vi "Actor Core.vi"(8 "error in":errorcluster, 11 "New Event UI in":refnum<class "New Event UI.lvclass">) -> (0 "error out":errorcluster, 3 "Actor out":refnum<class "Actor.lvclass">)   [LabVIEW 2019, in "New Event UI.lvlib" / "New Event UI.lvclass"]
doc: "(<B>Filename</B>: Actor Framework.lvlib:Actor.lvclass:Actor Core.vi)\n\nReceives messages to the actor, reacts to them, and initiates any error handling that may shut the actor down.\n\nDescendant classes may override this VI to append parallel tasks for the actor to complete while it handles messages. Overrides use the Call Parent Method node."
uses:
  New Event UI.lvclass
  <vilib>/ActorFramework/Actor/Actor.lvclass
  UI Controller/UI Controller/UI Controller.lvclass
  UI Controller/UI Controller Messages/Create New Event Msg/Create New Event Msg.lvclass
  C:/GIT/Event-Diplom/Source/Event Diplom NI-AF/UI Controller/UI Controller/UI Controller.lvclass
  C:/Program Files (x86)/National Instruments/LabVIEW 2019/vi.lib/ActorFramework/Actor/Actor.lvclass
  <vilib>/ActorFramework/Stop Msg/Stop Msg.lvclass
  <vilib>/GPower/UI/Library/GP UI.lvlib
panel:
  in  "Cancel Button":bool
  in  "OK Button":bool
  in  "Member Data File Path":path
  in  "Description":string
  in  "Event Name":string
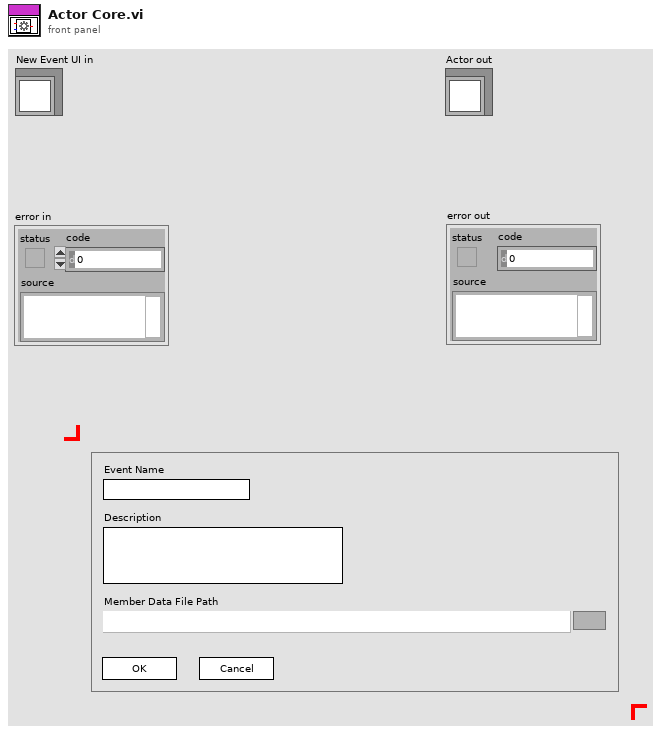
[diagram p1: front panel]
types:
  T1 = cluster{"Event Name":string, "Description":string, "Member Data File Path":path}
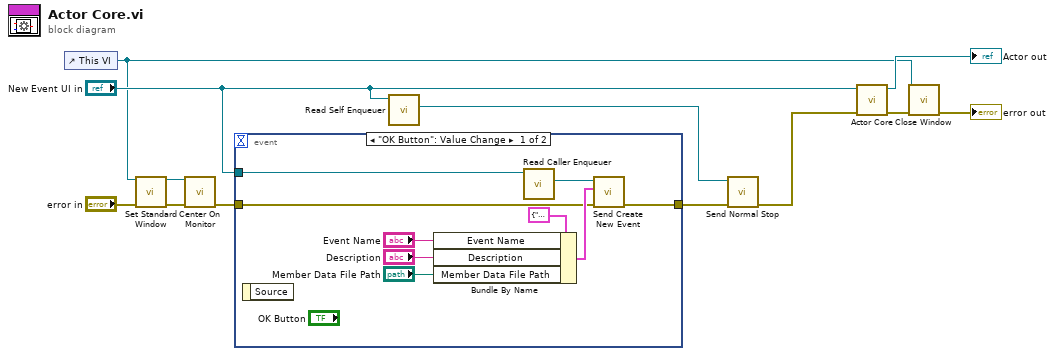
[diagram p0: block diagram]
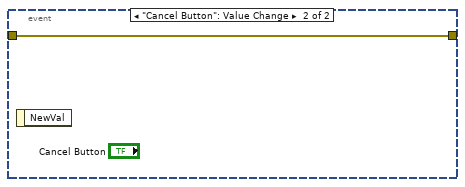
[diagram p2: hidden frame]
diagram:
  n1 = control-ref of="This VI"() -> (w3:refnum<vi>)
  n2 = call <vilib>:"Set Standard Window.vi"("VI Refnum"=w3, "Error in"="error in") -> ("Error out"=w6:errorcluster)  [unwired: 13 in]
  n3 = call <vilib>:"Center On Monitor.vi"("VI Refnum"=w3, "Error in"=w6) -> ("Error out"=w1:errorcluster)  [unwired: 13 in]
  n4 = event shown="[0] \"OK Button\": Value Change" {
    selector: _ -> [_ _]
    dyn-events: _ -> [_ _]
    timeout: _ -> [_ _]
    tunnel: "New Event UI in" -> [w20 _]
    tunnel: [w13 w21] -> w9
    tunnel: w1 -> [w12 w21]
    event "OK Button": Value Change {
      n5 = event-data() -> ()  [unwired: 1 in, 1 out]
      n6 = Bundle By Name(cluster=T1 {"Event Name"="", "Description"="", "Member Data File Path"=path ""} ("Event"), "Event Name"="Event Name", "Description"="Description", "Member Data File Path"="Member Data File Path") -> (w14:T1)
      n7 = call <vilib>:"Read Caller Enqueuer.vi"("Actor"=w20) -> ("Caller Enqueuer"=w19:refnum<class "Message Enqueuer.lvclass">)  [unwired: 10 in]
      n8 = call "Send Create New Event.vi"("error in (no error)"=w12, "Event"=w14, "Message Enqueuer"=w19) -> ("error out"=w13:errorcluster)  [unwired: 7 in, 1 out]
    }
    event "Cancel Button": Value Change {
      n9 = event-data() -> ()  [unwired: 1 in, 1 out]
    }
  }
  n10 = call <vilib>:"Read Self Enqueuer.vi"("Actor"="New Event UI in") -> ("Self Enqueuer"=w8:refnum<class "Message Enqueuer.lvclass">)  [unwired: 10 in]
  n11 = call <vilib>:"Send Normal Stop.vi"("error in (no error)"=w9, "Message Enqueuer"=w8) -> ("error out"=w7:errorcluster)  [unwired: 9 in]
  n12 = call-parent "Actor Core.vi"("error in"=w7, "UI Controller in"="New Event UI in") -> ("error out"=w5:errorcluster, "Actor out"=→"Actor out":refnum<class "Actor.lvclass">)  [unwired: 8 in]
  n13 = call <vilib>:"Close Window.vi"("VI Refnum"=w3, "Error in"=w5) -> ("Error out"=→"error out":errorcluster)  [unwired: 13 in]
